vi "linkCount.vi"(8 "error in (no error)":errorcluster, 10 "count in":u32, 11 "LLNode in":refnum<class "LLNode.lvclass">) -> (0 "error out":errorcluster, 2 "count out":u32, 3 "LLNode out":refnum<class "LLNode.lvclass">)   [LabVIEW 2009, in "LLNode.lvclass"]
uses:
  LLNode.lvclass
  Node/Node.lvclass
  LLNode.lvclass/LLNode.ctl
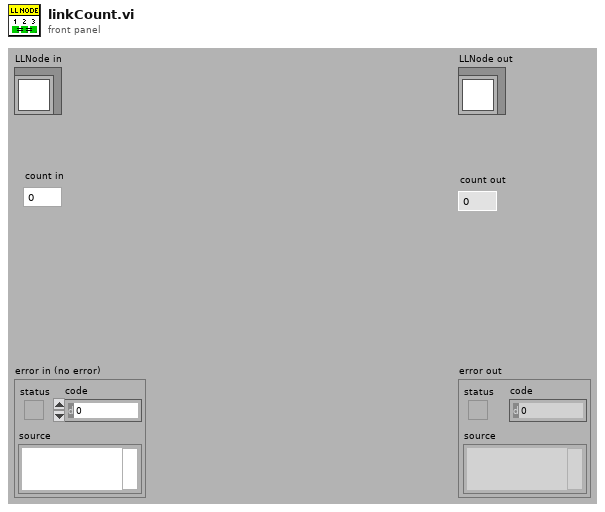
[diagram p1: front panel]
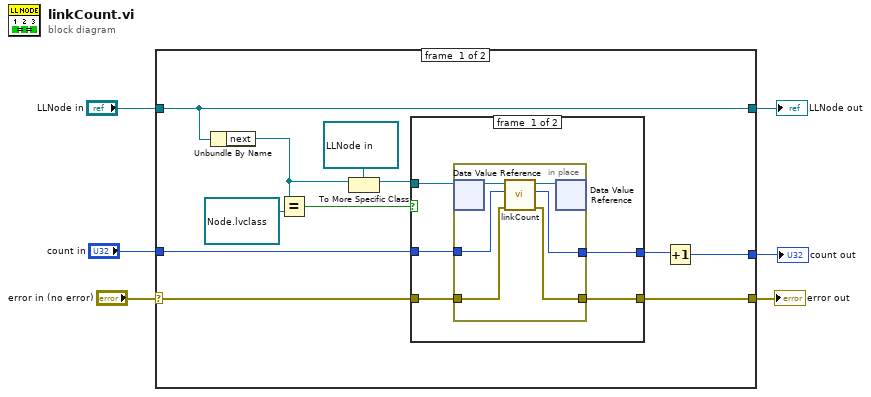
[diagram p0: block diagram]
diagram:
  n1 = case shown="No Error" "error in (no error)" {
    selector: "error in (no error)" -> [w10 w33]
    tunnel: [w7 w33] -> w5
    tunnel: [w14 w32] -> w3
    tunnel: "LLNode in" -> [w14 w32]
    tunnel: "count in" -> [w15 w31]
    tunnel: [w8 w31] -> w1
    frame #0 {
      n2 = Unbundle By Name(w14) -> ("next"=w11:refnum<data-value>)
      n3 = Equal?(x=w11, y=refnum<data-value> refnum) -> (x = y?=w16:bool)
      n4 = To More Specific Class(target class=refnum<data-value> refnum ("data value reference"), reference=w11) -> (specific class reference=w13:refnum<data-value>)  [unwired: 1 in, 1 out]
      n5 = case shown="False" w16 {
        tunnel: w15 -> [w20 w30]
        tunnel: [w19 w30] -> w9
        tunnel: w13 -> [w22 _]
        tunnel: w10 -> [w21 w29]
        tunnel: [w18 w29] -> w7
        frame #0 {
          n6 = in-place {
            in-place-border: w21 -> [w26]
            in-place-border: w20 -> [w25]
            in-place-border: [w24] -> w19
            in-place-border: [w23] -> w18
            n7 = in-place-dvr #1(w22) -> (w28:refnum<class "LLNode.lvclass">)  [unwired: 1 out]
            n8 = call "linkCount.vi"("error in (no error)"=w26, "count in"=w25, "LLNode in"=w28) -> ("error out"=w23:errorcluster, "count out"=w24:u32, "LLNode out"=w27:refnum<class "LLNode.lvclass">)  [unwired: 6 in]
            n9 = in-place-dvr #1(w27) -> ()  [unwired: 2 out]
          }
        }
        frame #1 {
        }
      }
      n10 = Increment(x=w9) -> (x+1=w8:u32)
    }
    frame #1 {
    }
  }
  "error out" <- w5
  "LLNode out" <- w3
  "count out" <- w1
